vi "Upload_To_ADAM_Server.vi"(1 "First Loop":bool, 2 "Averaging Period (s)":dbl=1.0, 3 "Shift In":dbl[](array[numeric]), 4 "Channel Values":dbl[](array[numeric]), 5 "Give Variance":bool, 6 "Channel Names":string[](array[string])) -> (0 "Shift Out":dbl[](array[numeric]))   [LabVIEW 2020]
uses:
  ADAM Controls/Update_scan_value.ctl
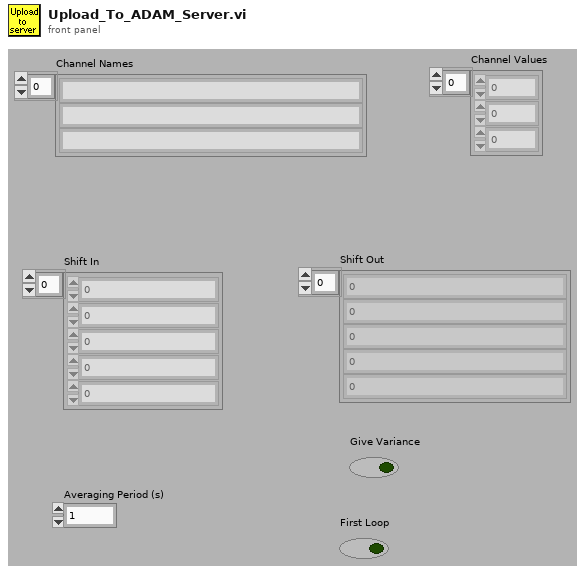
[diagram p1: front panel]
types:
  T1 = typedef "Update_scan_value.ctl" = cluster{"Channel Name":string, "New Value":dbl, "!Auto_Off":bool}
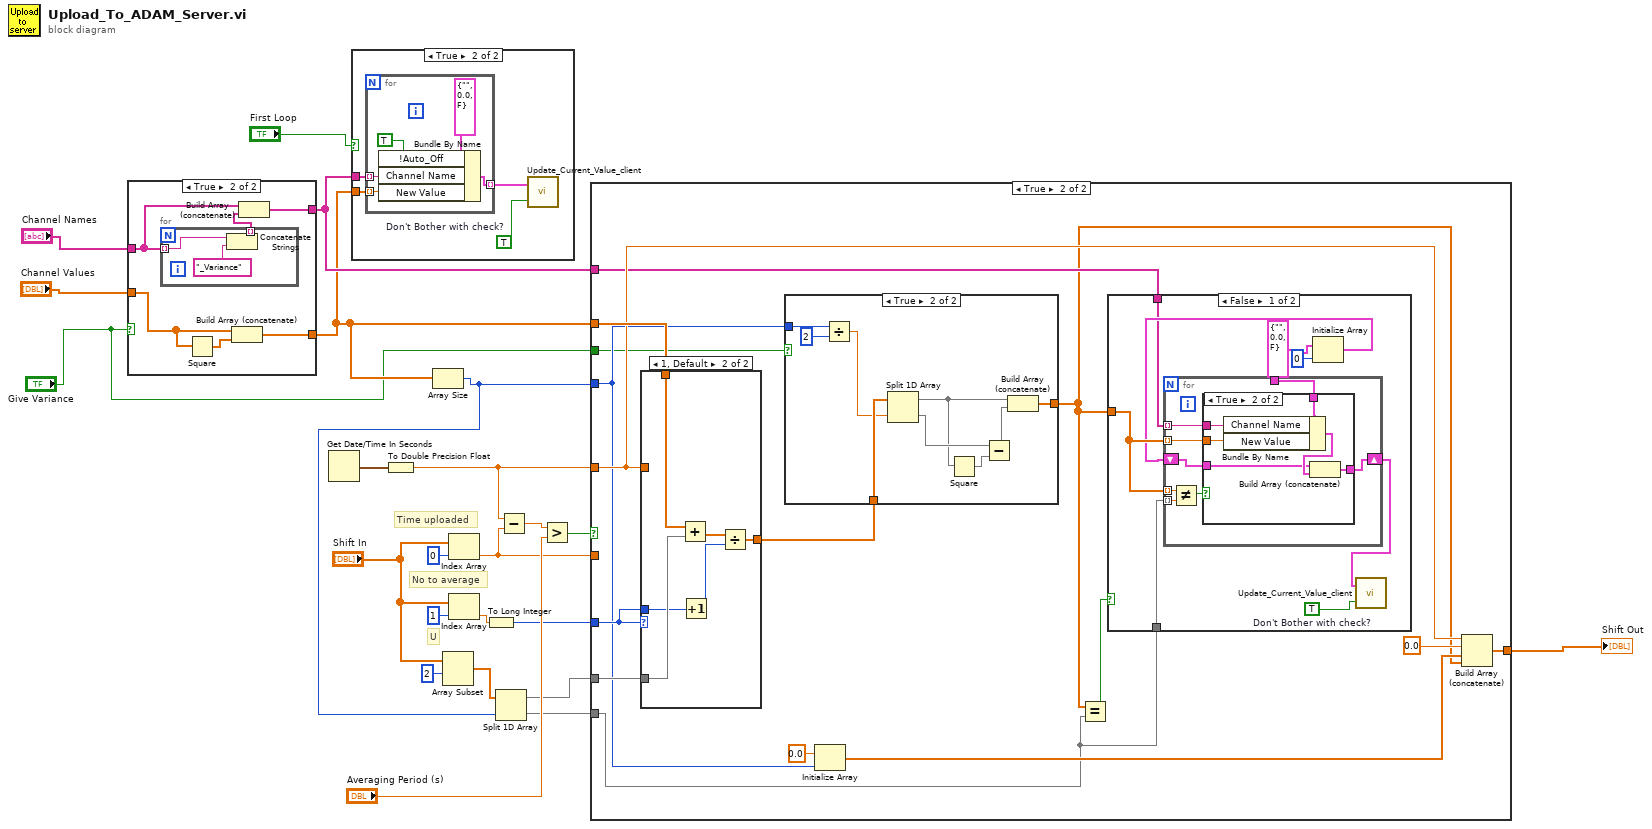
[diagram p0: block diagram]
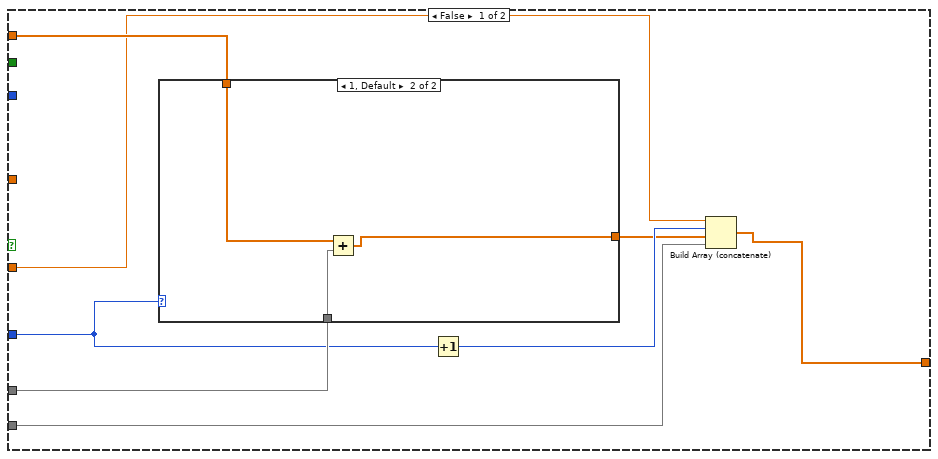
[diagram p4: hidden frame]
diagram:
  # "U"
  # "No to average"
  # "Time uploaded"
  n1 = case shown="True" "Give Variance" {
    tunnel: "Channel Names" -> [w25 w31]
    tunnel: [w25 w29] -> w4
    tunnel: "Channel Values" -> [w24 w27]
    tunnel: [w24 w26] -> w2
    frame False {
    }
    frame True {
      n2 = for {
        tunnel: w31 -> [w33] mode=indexing
        tunnel: [w32] -> w30 mode=indexing
        n3 = Concatenate Strings(w33, "_Variance") -> (w32:string)
      }
      n4 = Square(x=w27) -> (x^2=w28:dbl[])
      n5 = Build Array (concatenate)(w27, w28) -> (w26:dbl[])
      n6 = Build Array (concatenate)(w31, w30) -> (w29:string[])
    }
  }
  n7 = Get Date/Time In Seconds() -> (seconds since 1Jan1904=w22:timestamp)
  n8 = case shown="True" "First Loop" {
    tunnel: w4 -> [_ w36]
    tunnel: w2 -> [_ w35]
    frame False {
    }
    frame True {
      w38 = TRUE  # Don't Bother with check?
      n9 = for {
        tunnel: [w42] -> w37 mode=indexing
        tunnel: w36 -> [w41] mode=indexing
        tunnel: w35 -> [w40] mode=indexing
        n10 = Bundle By Name(cluster=T1 {"Channel Name"="", "New Value"=0.0, "!Auto_Off"=FALSE} ("Update Scan Value Cluster"), "!Auto_Off"=TRUE, "Channel Name"=w41, "New Value"=w40) -> (w42:T1)
      }
      n11 = call "Update_Current_Value_client.vi"("Don't Bother with check?"=w38, "Update array in"=w37) -> ()
    }
  }
  n12 = To Double Precision Float(number=w22) -> (double precision float=w13:dbl)
  n13 = Array Size(array=w2) -> (size(s)=w9:i32)
  n14 = Array Subset(array="Shift In", index=2) -> (w10:dbl[])  [unwired: 1 in]
  n15 = Index Array(array="Shift In", index=0) -> (element=w11:dbl)
  n16 = Index Array(array="Shift In", index=1) -> (element=w15:dbl)
  n17 = To Long Integer(number=w15) -> (32bit integer=w14:i32)
  n18 = Split 1D Array(array=w10, index=w9) -> (first subarray=w8:dbl[], second subarray=w7:dbl[])
  n19 = Subtract(x=w13, y=w11) -> (x-y=w21:dbl)
  n20 = Greater?(x=w21, y="Averaging Period (s)") -> (0:w19:bool)
  n21 = case shown="True" w19 {
    tunnel: w2 -> [w51 w70]
    tunnel: w8 -> [w50 w65]
    tunnel: w14 -> [w48 w69]
    tunnel: w13 -> [_ w68]
    tunnel: [w45 w66] -> w12
    tunnel: w11 -> [w49 _]
    tunnel: w9 -> [_ w59]
    tunnel: w7 -> [w44 w61]
    tunnel: w4 -> [_ w60]
    tunnel: "Give Variance" -> [_ w56]
    frame False {
      n22 = case shown="1, Default" w48 {
        tunnel: w51 -> [w52 w55]
        tunnel: w50 -> [_ w54]
        tunnel: [w52 w53] -> w46
        frame 0 {
        }
        frame 1, Default {
          n23 = Add(x=w55, y=w54) -> (x+y=w53:dbl[])
        }
      }
      n24 = Increment(x=w48) -> (x+1=w47:i32)
      n25 = Build Array (concatenate)(w49, w47, w46, w44) -> (w45:dbl[])
    }
    frame True {
      n26 = case shown="1, Default" w69 {
        tunnel: w68 -> [_ _]
        tunnel: w65 -> [_ w109]
        tunnel: w70 -> [w104 w110]
        tunnel: w69 -> [_ w108]
        tunnel: [w104 w105] -> w58
        frame 0 {
        }
        frame 1, Default {
          n27 = Add(x=w110, y=w109) -> (x+y=w107:dbl[])
          n28 = Increment(x=w108) -> (x+1=w106:i32)
          n29 = Divide(x=w107, y=w106) -> (x/y=w105:dbl[])
        }
      }
      n30 = case shown="True" w56 {
        tunnel: w59 -> [_ w80]
        tunnel: w58 -> [w71 w78]
        tunnel: [w71 w73] -> w57
        frame False {
        }
        frame True {
          n31 = Divide(x=w80, y=2) -> (x/y=w77:dbl)
          n32 = Split 1D Array(array=w78, index=w77) -> (first subarray=w75:dbl[], second subarray=w76:dbl[])
          n33 = Square(x=w75) -> (x^2=w72:dbl[])
          n34 = Subtract(x=w76, y=w72) -> (x-y=w74:dbl[])
          n35 = Build Array (concatenate)(w75, w74) -> (w73:dbl[])
        }
      }
      n36 = Initialize Array(0.0 ("element"), w59) -> (w63:dbl[])
      n37 = Equal?(x=w57, y=w61) -> (x = y?=w62:bool)
      n38 = case shown="False" w62 {
        tunnel: w57 -> [w87 _]
        tunnel: w61 -> [w86 _]
        tunnel: w60 -> [w81 _]
        frame False {
          w88 = TRUE  # Don't Bother with check?
          w85 = T1 {"Channel Name"="", "New Value"=0.0, "!Auto_Off"=FALSE} ("Update Scan Value Cluster")
          n39 = Initialize Array(w85, 0 ("dimension size")) -> (w83:T1[])
          n40 = for {
            tunnel: w85 -> [w96]
            tunnel: w81 -> [w95] mode=indexing
            tunnel: w87 -> [w94] mode=indexing
            shift-right: [w90] -> w82
            shift-left: w83 -> [w91]
            tunnel: w87 -> [w93] mode=indexing
            tunnel: w86 -> [w92] mode=indexing
            n41 = Not Equal?(x=w93, y=w92) -> (x != y?=w89:bool)
            n42 = case shown="True" w89 {
              tunnel: w96 -> [_ w103]
              tunnel: w95 -> [_ w102]
              tunnel: w94 -> [_ w101]
              tunnel: w91 -> [w97 w99]
              tunnel: [w97 w98] -> w90
              frame False {
              }
              frame True {
                n43 = Bundle By Name(cluster=w103, "Channel Name"=w102, "New Value"=w101) -> (w100:T1)
                n44 = Build Array (concatenate)(w99, w100) -> (w98:T1[])
              }
            }
          }
          n45 = call "Update_Current_Value_client.vi"("Don't Bother with check?"=w88, "Update array in"=w82) -> ()
        }
        frame True {
        }
      }
      n46 = Build Array (concatenate)(w68, 0.0 ("element"), w63, w57) -> (w66:dbl[])
    }
  }
  "Shift Out" <- w12
